vi "TDMS_READ.vi"() -> ()   [LabVIEW 2021]
panel:
  out "Secante Y Cosecante":waveform(dbl)[](graph)
  out "Tangente Y Cotangente":waveform(dbl)[](graph)
  out "Seno Y Coseno":waveform(dbl)[](graph)
  in  "File Path 2":path
  # "Mendoza Meza Manuel Everardo"
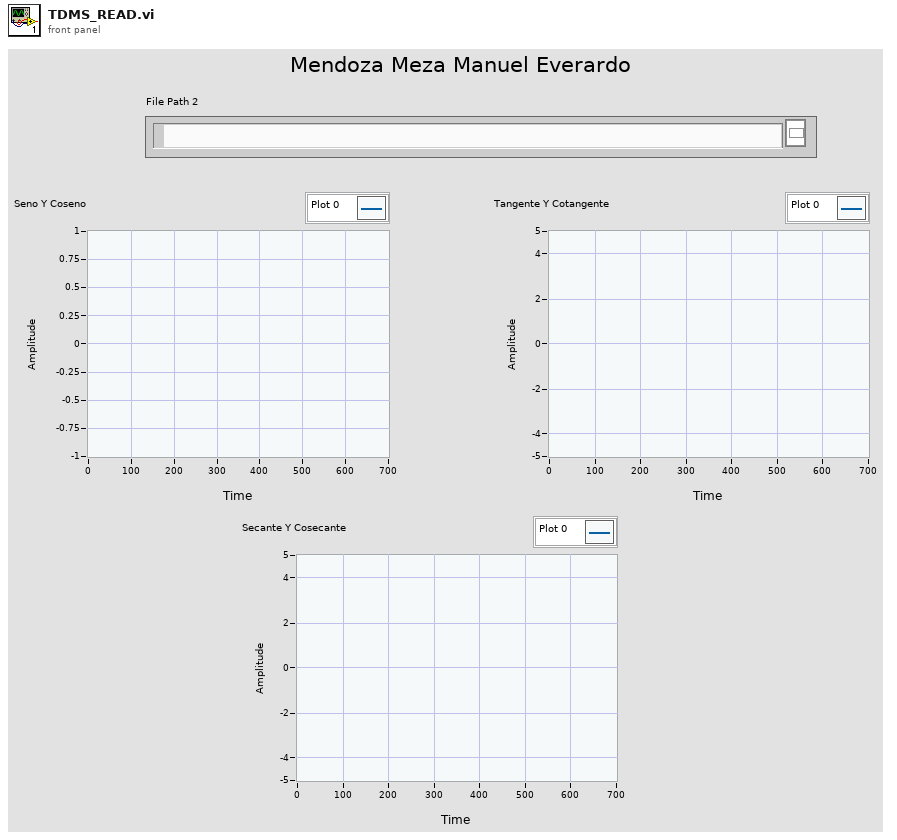
[diagram p1: front panel]
types:
  T1 = enum16{"open", "open or create", "create or replace", "create", "open (read-only)"}
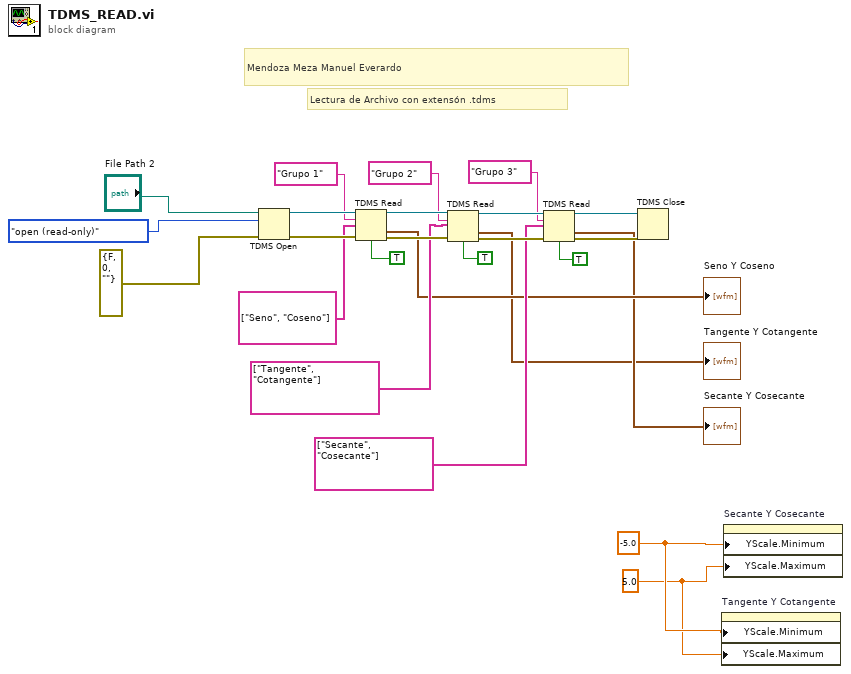
[diagram p0: block diagram]
diagram:
  w1 = 5.0 ("Y Scale.Range:Maximum")
  w2 = -5.0 ("Y Scale.Range:Minimum")
  # "Lectura de Archivo con extensón .tdms"
  # "Mendoza Meza Manuel Everardo"
  n1 = TDMS Open(8:errorcluster {"status"=FALSE, "code"=0, "source"=""} ("error in (no error)"), 10:T1."open (read-only)" ("operation (0:open)"), 11:"File Path 2") -> (0:w21:errorcluster, 3:w22:refnum<k34>)  [unwired: 4 in]
  n2 = TDMS Read(0:w22, 5:"Grupo 1" ("group name in (Untitled)"), 7:string[] ["Seno", "Coseno"] ("channel name(s) in (Untitled)"), 11:w21, 13:TRUE ("return channels in file order? (F)")) -> (4:w17:refnum<k34>, 10:→"Seno Y Coseno":waveform(dbl)[], 15:w20:errorcluster)  [unwired: 3 in, 3 out]
  n3 = TDMS Read(0:w17, 5:"Grupo 2" ("group name in (Untitled)"), 7:string[] ["Tangente", "Cotangente"] ("channel name(s) in (Untitled)"), 11:w20, 13:TRUE ("return channels in file order? (F)")) -> (4:w16:refnum<k34>, 10:→"Tangente Y Cotangente":waveform(dbl)[], 15:w19:errorcluster)  [unwired: 3 in, 3 out]
  n4 = TDMS Read(0:w16, 5:"Grupo 3" ("group name in (Untitled)"), 7:string[] ["Secante", "Cosecante"] ("channel name(s) in (Untitled)"), 11:w19, 13:TRUE ("return channels in file order? (F)")) -> (4:w15:refnum<k34>, 10:→"Secante Y Cosecante":waveform(dbl)[], 15:w18:errorcluster)  [unwired: 3 in, 3 out]
  n5 = TDMS Close(8:w18, 11:w15) -> ()  [unwired: 2 out]
  n6 = property on="Tangente Y Cotangente" class="WFGraph (strict)"("YScale.Minimum"=w2, "YScale.Maximum"=w1) -> ()  [unwired: 2 in, 2 out]
  n7 = property on="Secante Y Cosecante" class="WFGraph (strict)"("YScale.Minimum"=w2, "YScale.Maximum"=w1) -> ()  [unwired: 2 in, 2 out]
